vi "Create Transfer Group (old).vi"(4 "engine offset":u64, 5 "Debug Flags":refnum<class "Debug Flags.lvclass">, 6 "plugin id":i32, 7 "framework id":i32, 8 "error in (no error)":errorcluster, 9 "Direction":T1, 10 "Timing":refnum<class "Transfer Group Timing.lvclass">, 11 "Transfers":refnum<class "Transfer.lvclass">[](array[class])) -> (0 "error out":errorcluster, 3 "Transfer Group out":refnum<class "Transfer Group.lvclass">)   [LabVIEW 2017, in "DSF Core.lvlib" / "Transfer Group.lvclass"]
uses:
  Transfer Group.lvclass
  Transfer/Transfer.lvclass
  Timing/Transfer Group Timing.lvclass
  DSF Configuration API/Public/Controls/DSF Direction.ctl
  Debug/Debug Flags/Debug Flags.lvclass
  Transfer Group.lvclass/Transfer Group.ctl
  DSF Core.lvlib
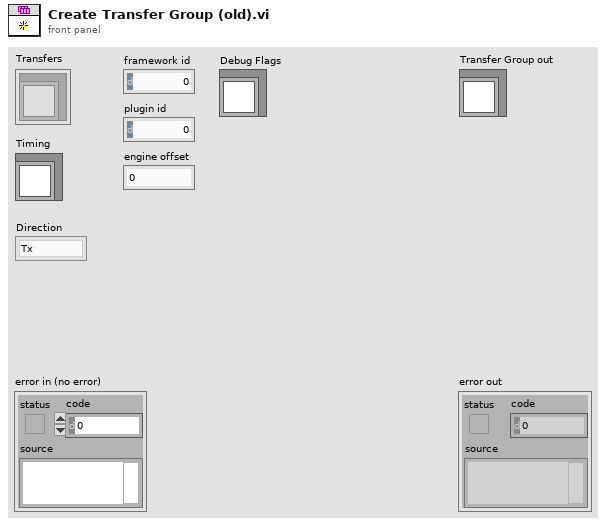
[diagram p1: front panel]
types:
  T1 = typedef "DSF Core.lvlib/DSF Direction.ctl" = enum8{"Tx", "Rx"}
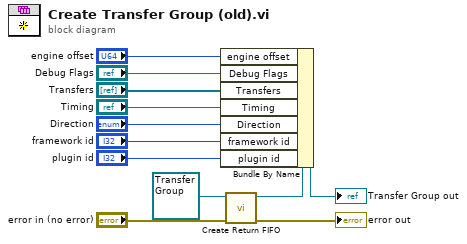
[diagram p0: block diagram]
diagram:
  n1 = call "Create Return FIFO.vi"("error in (no error)"="error in (no error)", "Transfer Group in"=refnum<class "Transfer Group.lvclass"> refnum ("Transfer Group type")) -> ("error out"=→"error out":errorcluster, "Transfer Group out"=w9:refnum<class "Transfer Group.lvclass">)  [unwired: 7 in, 1 out]
  n2 = Bundle By Name(cluster=w9, "engine offset"="engine offset", "Debug Flags"="Debug Flags", "Transfers"="Transfers", "Timing"="Timing", "Direction"="Direction", "framework id"="framework id", "plugin id"="plugin id") -> (→"Transfer Group out":refnum<class "Transfer Group.lvclass">)
